vi "PSAE_VCH_Quick Menu.vi"(8 "Error In (no error)":errorcluster, 9 "Menu Ref":refnum<k9>, 10 "Coords":T1, 11 "TreeRef":refnum<vi>) -> (0 "Error Out":errorcluster)   [LabVIEW 2016]
uses:
  <vilib>/Utility/miscctls.llb/LVMenuShortCut.ctl
  <vilib>/Utility/miscctls.llb/LVPoint32TypeDef.ctl
panel:
  # "Data Out"
  # "Data In"
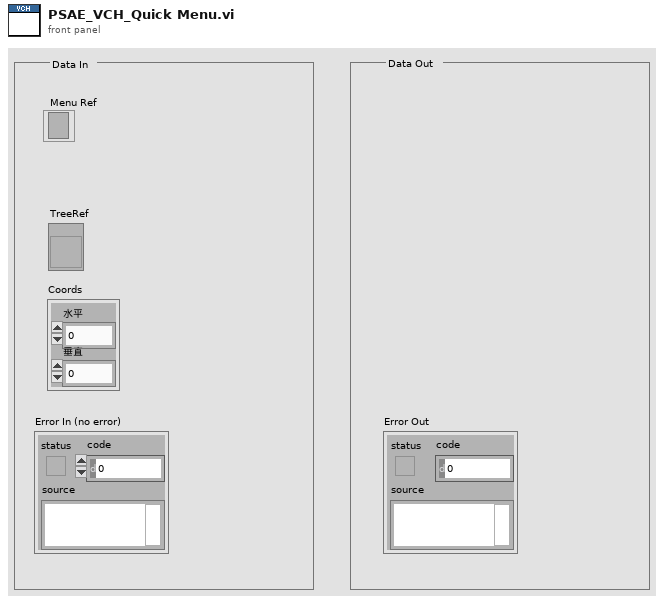
[diagram p1: front panel]
types:
  T1 = typedef "LVPoint32TypeDef.ctl" = cluster{"Horizontal":i32, "Vertical":i32}
  T2 = typedef "LVMenuShortCut.ctl" = cluster{"Include Shift Key?":bool, "Include Ctrl Key?":bool, "Shortcut Key":string}
  T3 = cluster{"Parent Tag":string, "Items":cluster{"Tag":string, "Name":string, "Enabled":bool, "Checked":bool, "Short Cut":T2}[]}[]
  T4 = cluster{"Tag":string, "Name":string, "Enabled":bool, "Checked":bool, "Short Cut":T2}[]
  T5 = cluster{"Tag":string, "Name":string, "Enabled":bool, "Checked":bool, "Short Cut":T2}
  T6 = cluster{"Parent Tag":string, "Items":cluster{"Tag":string, "Name":string, "Enabled":bool, "Checked":bool, "Short Cut":T2}[]}
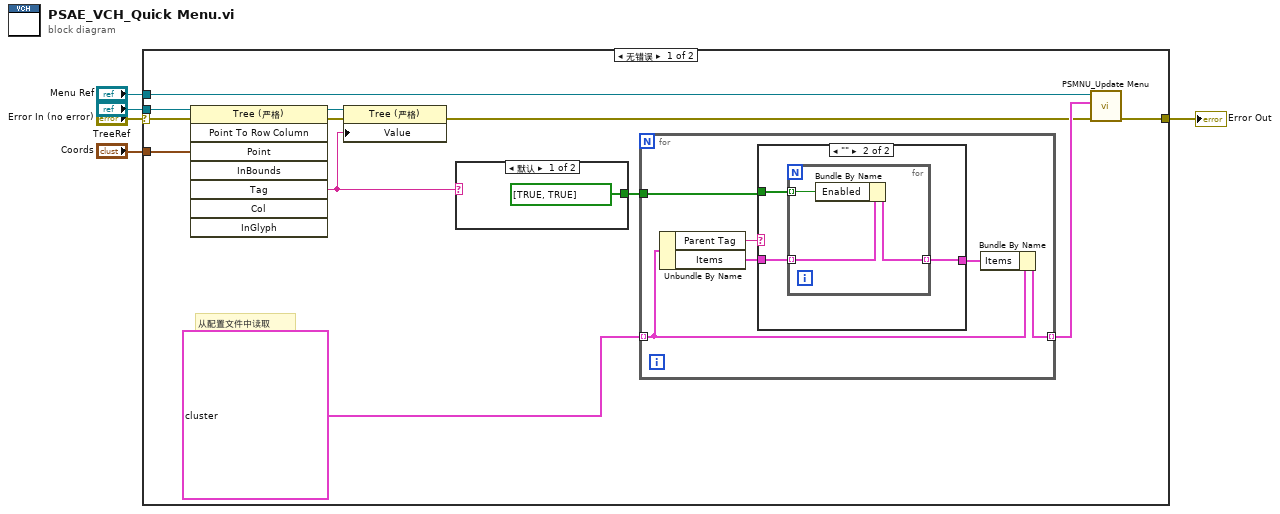
[diagram p0: block diagram]
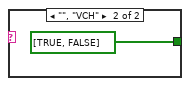
[diagram p2: hidden frame]
diagram:
  n1 = case shown="无错误" "Error In (no error)" {
    selector: "Error In (no error)" -> [w15 w33]
    tunnel: "Coords" -> [w17 _]
    tunnel: "TreeRef" -> [w16 _]
    tunnel: [w14 w33] -> w3
    tunnel: "Menu Ref" -> [w13 _]
    frame No Error {
      # "从配置文件中读取"
      n2 = invoke class="Tree (严格)" method="Point To Row Column"(reference=w16, error in=w15, "Point"=w17) -> (reference out=w9:refnum<vi>, error out=w8:errorcluster, "Tag"=w6:string)  [unwired: 5 in, 5 out]
      n3 = property class="Tree (严格)"(reference=w9, error in=w8, "Value"=w6) -> (error out=w7:errorcluster)  [unwired: 1 out]
      n4 = case shown="默认" w6 {
        tunnel: [bool[] [TRUE, TRUE] bool[] [TRUE, FALSE]] -> w11
        frame Default {
        }
        frame "", "VCH" {
        }
      }
      n5 = for {
        tunnel: T3 [{"Parent Tag"="", "Items"=[{"Tag"="添加", "Name"="Add", "Enabled"=TRUE, "Checked"=FALSE, "Short Cut"={"Include Shift Key?"=FALSE, "Include Ctrl Key?"=FALSE, "Shortcut Key"=""}}, {"Tag"="Delete", "Name"="删除", "Enabled"=TRUE, "Checked"=FALSE, "Short Cut"={"Include Shift Key?"=FALSE, "Include Ctrl Key?"=FALSE, "Shortcut Key"=""}}]}] ("Menu Items") -> [w22] mode=indexing
        tunnel: w11 -> [w23]
        tunnel: [w20] -> w10 mode=indexing
        n6 = Unbundle By Name(w22) -> ("Parent Tag"=w25:string, "Items"=w24:T4)
        n7 = case shown="\"\"" w25 {
          tunnel: w24 -> [w26 w29]
          tunnel: w23 -> [_ w28]
          tunnel: [w26 w27] -> w21
          frame Default {
          }
          frame "" {
            n8 = for {
              tunnel: w29 -> [w32] mode=indexing
              tunnel: [w31] -> w27 mode=indexing
              tunnel: w28 -> [w30] mode=indexing
              n9 = Bundle By Name(cluster=w32, "Enabled"=w30) -> (w31:T5)
            }
          }
        }
        n10 = Bundle By Name(cluster=w22, "Items"=w21) -> (w20:T6)
      }
      n11 = call <vilib>:"PSMNU_Update Menu.vi"("error in"=w7, "Menu Items"=w10, "Menu Ref"=w13) -> ("error out"=w14:errorcluster)  [unwired: 8 in]
    }
    frame Error {
    }
  }
  "Error Out" <- w3
